vi "Initial Matrix.vi"   [LabVIEW 2020, in "NI_AALBase.lvlib"]
uses:
  <vilib>/Analysis/NI_AALBase.lvlib
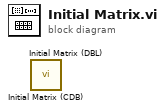
[diagram p0: block diagram]
diagram:
  n1 = call <vilib>:"Initial Matrix (CDB).vi"() -> ()  [unwired: 10 in, 2 out]
  n2 = call <vilib>:"Initial Matrix (DBL).vi"() -> ()  [unwired: 10 in, 2 out]
